vi "Create Variable Engine.vi"(8 "error in (no error)":errorcluster, 11 "Application in":refnum<class "Application.lvclass">) -> (0 "error out":errorcluster, 3 "Application out":refnum<class "Application.lvclass">)   [LabVIEW 2017, in "Application.lvlib" / "Application.lvclass"]
uses:
  Application.lvclass
  <vilib>/TSS/ACRObat Test Framework/Classes/Variable Engine/Class/Variable Engine.lvclass
  C:/Test System Services/Acrobat Framework/ACRObat Test Framework/Main Framework/Release/Test Framework/Classes/Base Objects/Base Class/Base Class/Base Class.lvclass
  Application.lvclass/Application.ctl
  Properties/App Properties.lvclass/App Properties.ctl
  <vilib>/TSS/ACRObat Test Framework/Classes/Base Objects/Base Class/Base Class/Base Class.lvclass
  Properties/App Properties.lvclass
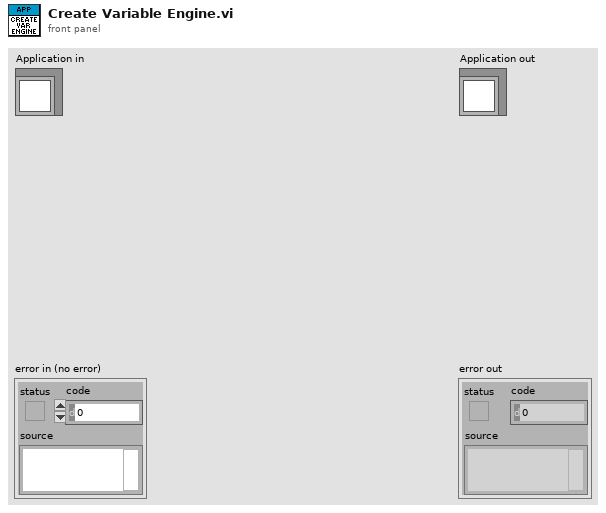
[diagram p1: front panel]
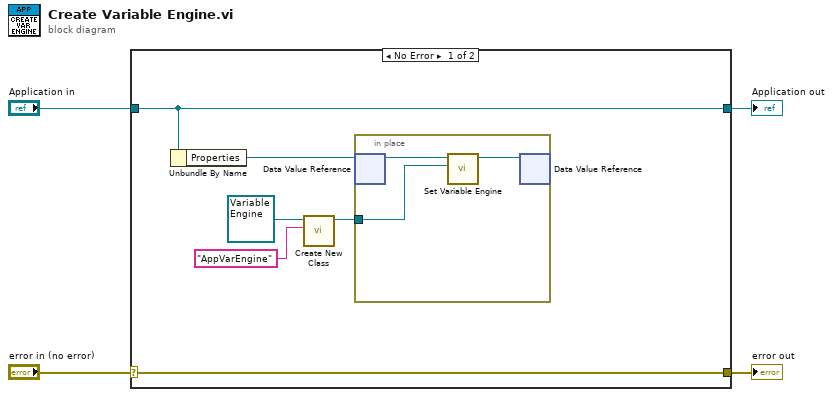
[diagram p0: block diagram]
diagram:
  n1 = case shown="No Error" "error in (no error)" {
    selector: "error in (no error)" -> [w10 w15]
    tunnel: [w10 w15] -> w3
    tunnel: [w9 w14] -> w1
    tunnel: "Application in" -> [w9 w14]
    frame No Error {
      n2 = Unbundle By Name(w9) -> ("Properties"=w8:refnum<data-value>)
      n3 = call <vilib>:"Create New Class.vi"("Name"="AppVarEngine", "Base Class in"=refnum<class "Variable Engine.lvclass"> refnum ("Variable Engine")) -> ("Base Class out"=w5:refnum<class "Variable Engine.lvclass">)  [unwired: 8 in, 1 out]
      n4 = in-place {
        in-place-border: w5 -> [w11]
        n5 = in-place-dvr #1(w8) -> (w13:refnum<class "App Properties.lvclass">)  [unwired: 1 out]
        n6 = call "Set Variable Engine.vi"("Variable Engine"=w11, "App Properties in"=w13) -> ("App Properties out"=w12:refnum<class "App Properties.lvclass">)  [unwired: 8 in, 1 out]
        n7 = in-place-dvr #1(w12) -> ()  [unwired: 2 out]
      }
    }
    frame Error {
    }
  }
  "error out" <- w3
  "Application out" <- w1
